vi "PacketsError.vi"(9 "Index":i32, 10 "Libraries":string[](array[string]), 11 "Packets errors in":string[](array[string])) -> (3 "Packets errors out":string[](array[string]))   [LabVIEW 2019, in "ByteLVDevEnv.lvlib"]
uses:
  ByteLVDevEnv.lvlib
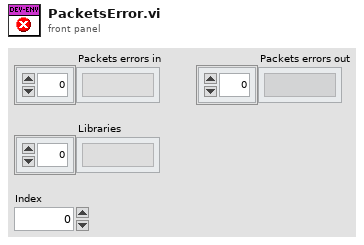
[diagram p1: front panel]
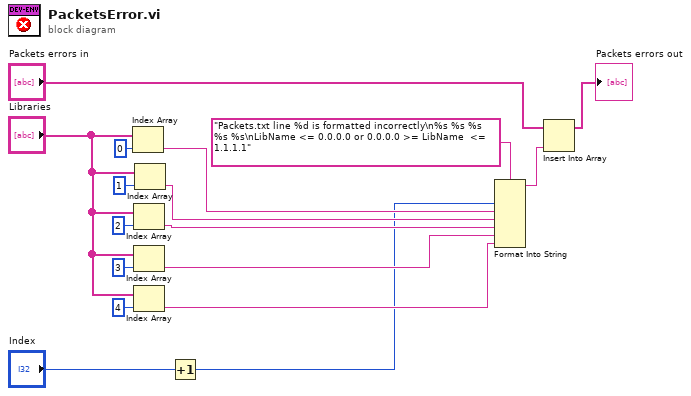
[diagram p0: block diagram]
diagram:
  n1 = Index Array(array="Libraries", index=0) -> (element=w12:string)
  n2 = Index Array(array="Libraries", index=2) -> (element=w14:string)
  n3 = Index Array(array="Libraries", index=3) -> (element=w15:string)
  n4 = Index Array(array="Libraries", index=4) -> (element=w16:string)
  n5 = Index Array(array="Libraries", index=1) -> (element=w13:string)
  n6 = Increment(x="Index") -> (x+1=w11:i32)
  n7 = Format Into String(format string="Packets.txt line %d is formatted incorrectly\n%s %s %s %s %s\nLibName <= 0.0.0.0 or 0.0.0.0 >= LibName  <= 1.1.1.1" ("string"), w11, w12, w13, w14, w15, w16) -> (resulting string=w17:string)  [unwired: 2 in, 1 out]
  n8 = Insert Into Array(array="Packets errors in", new element=w17) -> (→"Packets errors out":string[])  [unwired: 1 in]
